vi "initialize.vi"(0 "HGF_SVMonitor in":refnum<class "HGF_SVMonitor.lvclass">, 3 "initializationData":variant, 5 "error in (no error)":errorcluster, 7 "binaryString":string, 8 "I8 Array":i8[](array[numeric]), 9 "prependSize? (T)":bool, 11 "byteOrder (0:big-endian, network order)":T1(ring)) -> (14 "HGF_SVMonitor out":refnum<class "HGF_SVMonitor.lvclass">, 17 "found?":bool, 19 "error out":errorcluster)   [LabVIEW 2012, in "HGF_SV.lvlib" / "HGF_SVMonitor.lvclass"]
uses:
  HGF_SVMonitor.lvclass
  HGF_Monitor/HGF_Monitor.lvclass
  HGF_SVMonitor.lvclass/HGF_SVMonitor.ctl
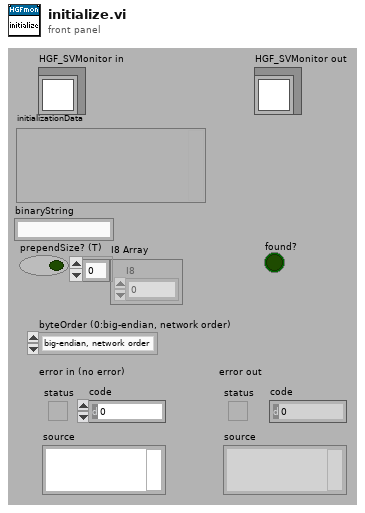
[diagram p1: front panel]
types:
  T1 = enum16{"big-endian, network order", "native, host order", "little-endian"}
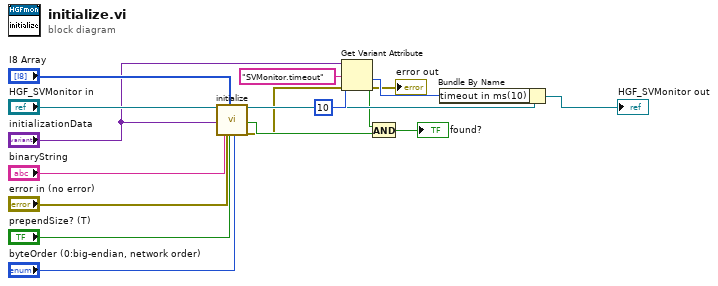
[diagram p0: block diagram]
diagram:
  n1 = call-parent "initialize.vi"("HGF_Base"="HGF_SVMonitor in", "initializationData"="initializationData", "error in (no error)"="error in (no error)", "binaryString"="binaryString", "I8 Array"="I8 Array", "prependSize? (T)"="prependSize? (T)", "byteOrder (0:big-endian, network order)"="byteOrder (0:big-endian, network order)") -> ("dup HGF_Base"=w13:refnum<class "HGF_SVMonitor.lvclass">, "found?"=w5:bool, "error out"=w3:errorcluster)  [unwired: 10 out]
  n2 = Get Variant Attribute(Variant="initializationData", name="SVMonitor.timeout", default value (empty Variant)=10 ("timeout in ms(10)"), error in=w3) -> (found=w1:bool, value=w14:i32, error out=→"error out":errorcluster)  [unwired: 1 out]
  n3 = And(x=w1, y=w5) -> (x .and. y?=→"found?":bool)
  n4 = Bundle By Name(cluster=w13, "timeout in ms(10)"=w14) -> (→"HGF_SVMonitor out":refnum<class "HGF_SVMonitor.lvclass">)
